vi "Initialize.vi"(8 "error in (no error)":errorcluster, 9 "Reset (T: Reset)":bool=TRUE, 10 "ID Query (T: Check)":bool=TRUE, 11 "Instrument Resource Name":refnum<visa-resource-name>) -> (0 "error out":errorcluster, 3 "dup VISA session":refnum<visa-resource-name>)   [LabVIEW 2018, in "Agilent PNA Series.lvlib"]
doc: "This VI passes the addressing information in the instrument descriptor to the Instr Open VI and returns the instrument ID. You can optionally reset the instrument by setting the front panel reset control. You must run this VI before using any of the instrument driver VIs for this instrument."
uses:
  Agilent PNA Series.lvlib
  <vilib>/regexp/Match Regular Expression.xnode
panel:
  # "(c) 2005-2015 National Instruments.  ALL RIGHTS RESERVED."
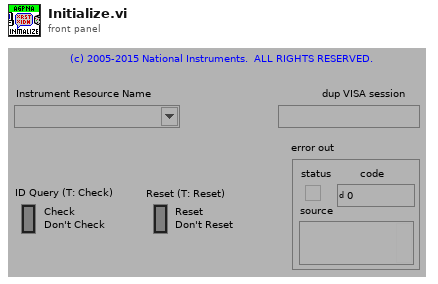
[diagram p1: front panel]
types:
  T1 = cluster{"Status":bool, "Code":i32, "Source (VI Name)":string}
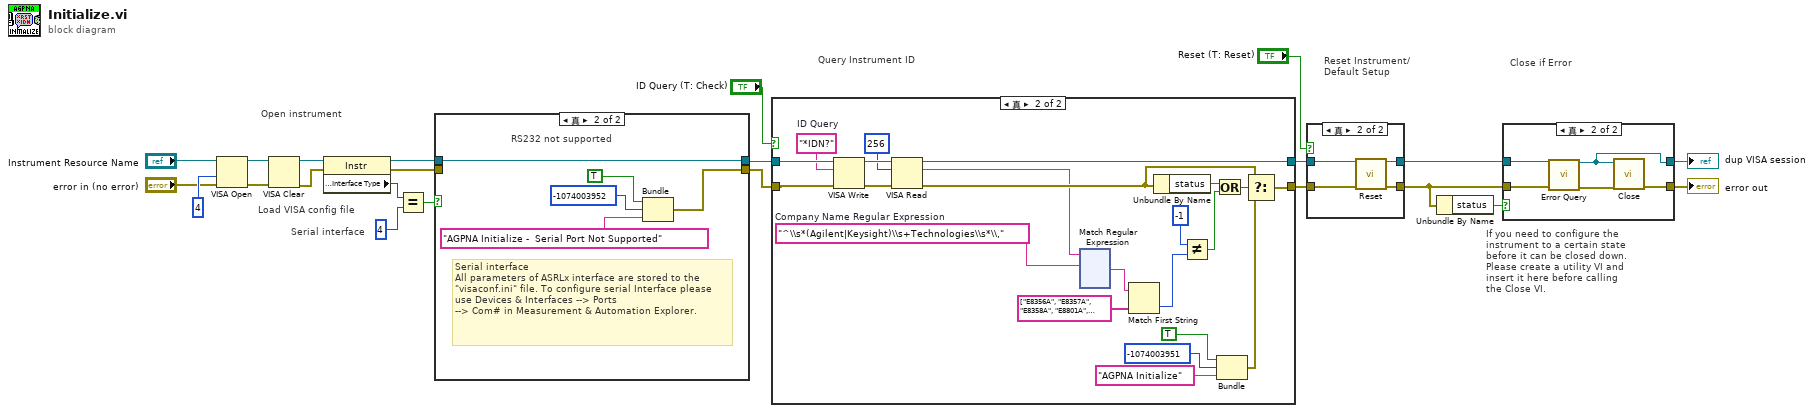
[diagram p0: block diagram]
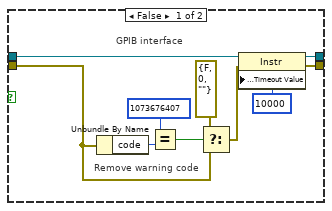
[diagram p2: hidden frame]
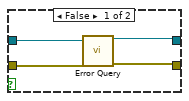
[diagram p3: hidden frame]
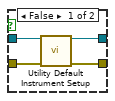
[diagram p4: hidden frame]
diagram:
  # "If you need to configure the \ninstrument to a certain state\nbefore it can be closed down. \nPlease create a utility VI and \ninsert it here before calling\nthe Close VI."
  # "Serial interface"
  # "Load VISA config file"
  # "Close if Error"
  # "Query Instrument ID"
  # "Reset Instrument/\nDefault Setup"
  # "Open instrument"
  n1 = VISA Open(access mode=u32 4, error in (no error)="error in (no error)", VISA resource name="Instrument Resource Name") -> (VISA resource name=w1:refnum<visa-resource-name>, error out=w2:errorcluster)  [unwired: 2 in]
  n2 = VISA Clear(VISA resource name=w1, error in (no error)=w2) -> (VISA resource name out=w4:refnum<visa-resource-name>, error out=w3:errorcluster)
  n3 = property class="Instr"(reference=w4, error in=w3) -> (reference out=w10:refnum<visa-resource-name>, error out=w11:errorcluster, "Interface Information:Interface Type"=w13:u16)
  n4 = Equal?(x=w13, y=u16 4) -> (x = y?=w12:bool)
  n5 = case shown="真" w12 {
    tunnel: w11 -> [w25 _]
    tunnel: w10 -> [w33 w34]
    tunnel: [w32 w35] -> w6
    tunnel: [w31 w34] -> w5
    frame False {
      # "Remove warning code"
      # "GPIB interface"
      n6 = Unbundle By Name(w25) -> ("code"=w26:i32)
      n7 = Equal?(x=1073676407, y=w26) -> (x = y?=w28:bool)
      n8 = Select(t=errorcluster {"status"=FALSE, "code"=0, "source"=""} ("error out"), s=w28, f=w25) -> (s? t:f=w24:errorcluster)
      n9 = property class="Instr"(reference=w33, error in=w24, "General Settings:Timeout Value"=u32 10000 ("Tmo Value")) -> (reference out=w31:refnum<visa-resource-name>, error out=w32:errorcluster)
    }
    frame True {
      # "RS232 not supported"
      # "Serial interface\nAll parameters of ASRLx interface are stored to the \"visaconf.ini\" file. To configure serial Interface please use Devices & Interfaces --> Ports \n--> Com# in Measurement & Automation Explorer."
      n10 = Bundle("Status"=TRUE, "Code"=-1074003952, "Source (VI Name)"="AGPNA Initialize -  Serial Port Not Supported") -> (w35:T1)  [unwired: 1 in]
    }
  }
  n11 = case shown="真" "ID Query (T: Check)" {
    tunnel: [w39 w62] -> w22
    tunnel: [w40 w59] -> w23
    tunnel: w5 -> [w40 w60]
    tunnel: w6 -> [w39 w61]
    frame False {
    }
    frame True {
      w41 = "^\\s*(Agilent|Keysight)\\s+Technologies\\s*\\,"  # Company Name Regular Expression
      w50 = "*IDN?"  # ID Query
      n12 = VISA Write(VISA resource name=w60, write buffer=w50, error in (no error)=w61) -> (VISA resource name out=w56:refnum<visa-resource-name>, error out=w54:errorcluster)  [unwired: 1 out]
      n13 = VISA Read(VISA resource name=w56, byte count=u32 256, error in (no error)=w54) -> (VISA resource name out=w59:refnum<visa-resource-name>, read buffer=w45:string, error out=w55:errorcluster)  [unwired: 1 out]
      n14 = xnode "Match Regular Expression"("输入字符串"=w45, "正则表达式"=w41) -> ("匹配之后"=w42:string)  [unwired: 4 in, 4 out]
      n15 = Match First String(2:string[] ["E8356A", "E8357A", "E8358A", "E8801A", "E8802A", "E8803A", "N3381A", "N3382A", "N3383A", "E8361A", "E8362A", "E8363A", "E8364A", "E8362B", "E8363B", "E8364B", "E5070A", "E5071A", "E5070B", "E5071B", "N5250A", "N5230A"] ("array"), 3:w42) -> (0:w44:i32)  [unwired: 1 out]
      n16 = Unbundle By Name(w55) -> ("status"=w52:bool)
      n17 = Not Equal?(x=-1, y=w44) -> (x != y?=w57:bool)
      n18 = Or(x=w52, y=w57) -> (x .or. y?=w53:bool)
      n19 = Bundle("Status"=TRUE, "Code"=-1074003951, "Source (VI Name)"="AGPNA Initialize") -> (w49:T1)  [unwired: 1 in]
      n20 = Select(t=w55, s=w53, f=w49) -> (s? t:f=w62:T1)
    }
  }
  n21 = case shown="真" "Reset (T: Reset)" {
    tunnel: w22 -> [w179 w181]
    tunnel: [w178 w184] -> w18
    tunnel: w23 -> [w180 w182]
    tunnel: [w177 w183] -> w17
    frame False {
      n22 = call "Utility Default Instrument Setup.vi"("VISA Resource Name"=w180, "error in (no error)"=w179) -> ("VISA Resource Name Out"=w177:refnum<visa-resource-name>, "error out"=w178:errorcluster)  [unwired: 12 in]
    }
    frame True {
      n23 = call "Reset.vi"("VISA Resource Name"=w182, "error in (no error)"=w181) -> ("VISA Resource Name Out"=w183:refnum<visa-resource-name>, "error out"=w184:errorcluster)  [unwired: 12 in]
    }
  }
  n24 = Unbundle By Name(w18) -> ("status"=w19:bool)
  n25 = case shown="真" w19 {
    tunnel: w17 -> [w188 w192]
    tunnel: w18 -> [w187 w191]
    tunnel: [w186 w189] -> w16
    tunnel: [w185 w193] -> w15
    frame False {
      n26 = call "Error Query.vi"("VISA Resource Name"=w188, "error in (no error)"=w187) -> ("VISA Resource Name Out"=w186:refnum<visa-resource-name>, "error out"=w185:errorcluster)  [unwired: 10 in, 2 out]
    }
    frame True {
      n27 = call "Error Query.vi"("VISA Resource Name"=w192, "error in (no error)"=w191) -> ("VISA Resource Name Out"=w189:refnum<visa-resource-name>, "error out"=w190:errorcluster)  [unwired: 10 in, 2 out]
      n28 = call "Close.vi"("Error In (no error)"=w190, "VISA Resource Name"=w189) -> ("Error Out"=w193:errorcluster)  [unwired: 9 in]
    }
  }
  "dup VISA session" <- w16
  "error out" <- w15
